vi "Create Measurement.vi"(8 "error in":errorcluster, 10 "measurement results":T3, 11 "measurement configuration":T2) -> (0 "error out":errorcluster, 3 "gRPCid out":T1)   [LabVIEW 2021, in "Measurement Client Template.lvlib"]
uses:
  Measurement Client Template.lvlib
  controls/Measurement Results.ctl
  controls/Measurement Configuration.ctl
  <vilib>/gRPC/LabVIEW gRPC Library/Shared/grpcId.ctl
  <vilib>/gRPC/Generated APIs/ni/measurementlink/discovery/v1/RPC Messages/ni_measurementlink_discovery_v1_ResolveServiceRequest.ctl
  <vilib>/Plug-In SDKs/Clients/Discovery V1/NI Discovery V1 Client.lvlib
  <vilib>/gRPC/Generated APIs/ni/measurementlink/discovery/v1/ni.measurementlink.discovery.v1.api.lvlib
  <vilib>/gRPC/LabVIEW gRPC Library/grpc-lvsupport-release.lvlib
  <vilib>/gRPC/Generated APIs/ni/measurementlink/measurement/v2/Measurement Service Client/Measurement Service Client.lvlib
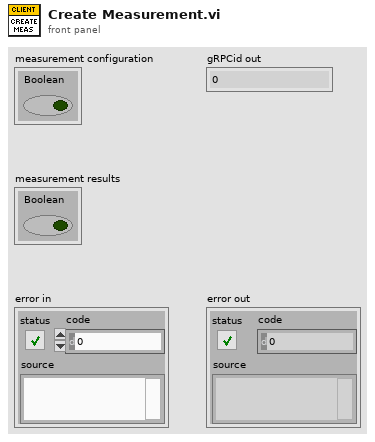
[diagram p1: front panel]
types:
  T1 = typedef "grpc-lvsupport-release.lvlib/grpcId.ctl" = u64
  T2 = typedef "Measurement Client Template.lvlib/Measurement Configuration.ctl" = cluster{"Boolean":bool}
  T3 = typedef "Measurement Client Template.lvlib/Measurement Results.ctl" = cluster{"Boolean":bool}
  T4 = typedef "ni.measurementlink.discovery.v1.api.lvlib/ni_measurementlink_discovery_v1_ResolveServiceRequest.ctl" = cluster{"provided_interface":string, "service_class":string}
  T5 = typedef "ni.measurementlink.discovery.v1.api.lvlib/ni_measurementlink_discovery_v1_ServiceLocation.ctl" = cluster{"location":string, "insecure_port":string, "ssl_authenticated_port":string}
  T6 = typedef "grpc-lvsupport-release.lvlib/Enum Metadata.ctl" = cluster{"Version":i32, "Name":string, "Type Url":string, "Enum Values":string, "Allow Alias":bool}
  T7 = typedef "grpc-lvsupport-release.lvlib/Message Metadata.ctl" = cluster{"Version":i32, "Name":string, "Type Url":string, "Elements":T8[], "Has Oneof":bool}
  T8 = typedef "grpc-lvsupport-release.lvlib/Message Element Metadata.ctl" = cluster{"Field Name":string, "Embedded Message Name":string, "Protobuf Index":i32, "MessageElementType":T9, "Repeated":bool, "Is in Oneof":bool, "Oneof Container Name":string}
  T9 = typedef "grpc-lvsupport-release.lvlib/Message Element Type.ctl" = enum32{"Int32Value", "FloatValue", "DoubleValue", "BoolValue", "StringValue", "MessageValue", "Int64Value", "UInt32Value", "UInt64Value", "EnumValue", "Bytes", "Fixed64", "Fixed32", "SFixed64", "SFixed32", "SInt64", "SInt32"}
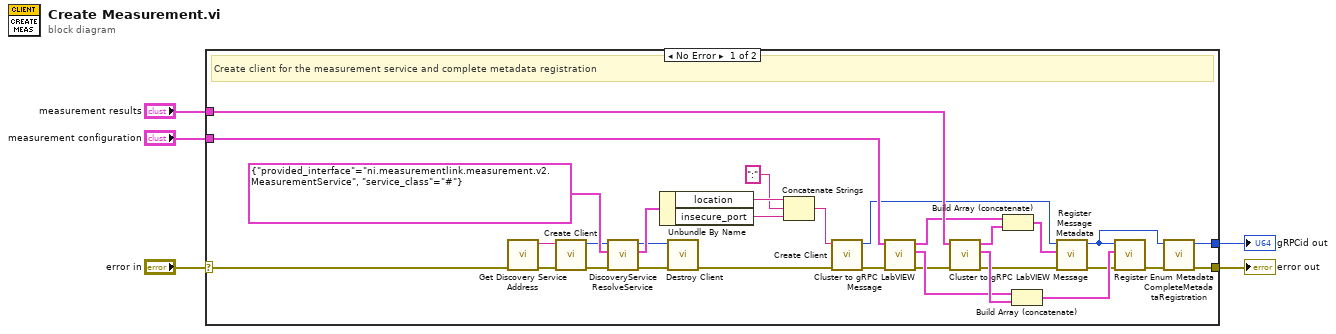
[diagram p0: block diagram]
diagram:
  n1 = case shown="No Error" "error in" {
    selector: "error in" -> [w33 w37]
    tunnel: "measurement results" -> [w22 _]
    tunnel: "measurement configuration" -> [w21 _]
    tunnel: [w15 w37] -> w2
    tunnel: [w14 _] -> w1
    frame No Error {
      # "Create client for the measurement service and complete metadata registration"
      n2 = call <vilib>:"Get Discovery Service Address.vi"("error in"=w33) -> ("error out"=w34:errorcluster, "address"=w35:string)  [unwired: 9 in]
      n3 = call <vilib>:"Create Client.vi"("error in"=w34, "address"=w35) -> ("error out"=w32:errorcluster, "gRPC ID Out"=w6:T1)  [unwired: 8 in]
      n4 = call <vilib>:"DiscoveryService ResolveService.vi"("error in"=w32, "Request Data"=T4 {"provided_interface"="ni.measurementlink.measurement.v2.MeasurementService", "service_class"="#"} ("resolve service request data"), "gRPC ID"=w6) -> ("error out"=w29:errorcluster, "Response Data"=w31:T5, "gRPC ID out"=w30:T1)  [unwired: 6 in]
      n5 = Unbundle By Name(w31) -> ("location"=w11:string, "insecure_port"=w10:string)
      n6 = call <vilib>:"Destroy Client.vi"("error in"=w29, "gRPC ID"=w30) -> ("error out"=w28:errorcluster)  [unwired: 9 in]
      n7 = Concatenate Strings(w11, ":" ("string"), w10) -> (w9:string)
      n8 = call <vilib>:"Create Client.vi"("error in"=w28, "address"=w9) -> ("error out"=w13:errorcluster, "gRPC ID Out"=w20:T1)  [unwired: 8 in]
      n9 = call <vilib>:"Cluster to gRPC LabVIEW Message.vi"("error in"=w13, "Cluster"=w21) -> ("error out"=w12:errorcluster, "gRPC Enum Metadata out"=w26:T6[], "gRPC Message Metadata []"=w19:T7[])  [unwired: 7 in]
      n10 = call <vilib>:"Cluster to gRPC LabVIEW Message.vi"("error in"=w12, "Cluster"=w22) -> ("error out"=w16:errorcluster, "gRPC Enum Metadata out"=w27:T6[], "gRPC Message Metadata []"=w17:T7[])  [unwired: 7 in]
      n11 = Build Array (concatenate)(w19, w17) -> (w18:T7[])
      n12 = Build Array (concatenate)(w26, w27) -> (w25:T6[])
      n13 = call <vilib>:"Register Message Metadata.vi"("error in"=w16, "Messages"=w18, "gRPCid in"=w20) -> ("error out"=w23:errorcluster, "gRPCid out"=w36:T1)  [unwired: 7 in]
      n14 = call <vilib>:"Register Enum Metadata.vi"("error in"=w23, "Enum Metadata"=w25, "gRPCid in"=w36) -> ("error out"=w24:errorcluster)  [unwired: 7 in, 1 out]
      n15 = call <vilib>:"CompleteMetadataRegistration.vi"("error in"=w24, "gRPC ID in"=w36) -> ("error out"=w15:errorcluster, "gRPC ID Out"=w14:T1)  [unwired: 8 in]
    }
    frame Error {
      # "Pass"
    }
  }
  "error out" <- w2
  "gRPCid out" <- w1
